vi "MCLScanPSD.vi"(0 "In Image":T1(plugin-control)=refnum, 1 "Trap Detector":dbl[](array[numeric]), 2 "Scan steps (x)":u64, 3 "Scan lines (y)":u64, 4 "Cycles/step (MCL)":u64, 5 "NewScan?":bool) -> (14 "Out Image":T1(plugin-control))   [LabVIEW 2013]
uses:
  <vilib>/Analysis/baseanly.llb/Mean (DBL).vi
  <vilib>/vision/NI_Vision_Development_Module.lvlib
  <vilib>/Analysis/NI_AALBase.lvlib
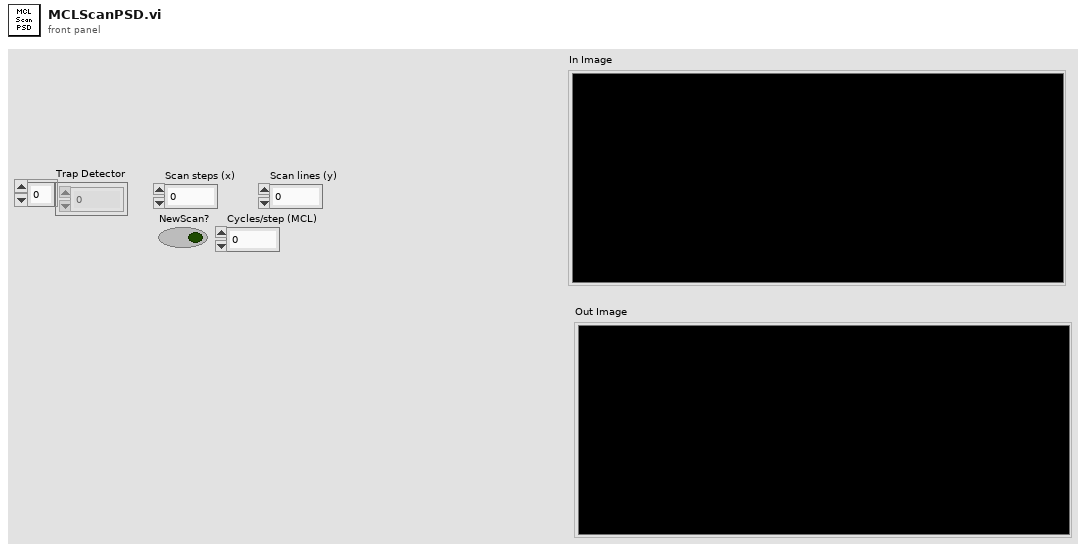
[diagram p1: front panel]
types:
  T1 = typedef "IMAQ Image.ctl" = refnum<image>
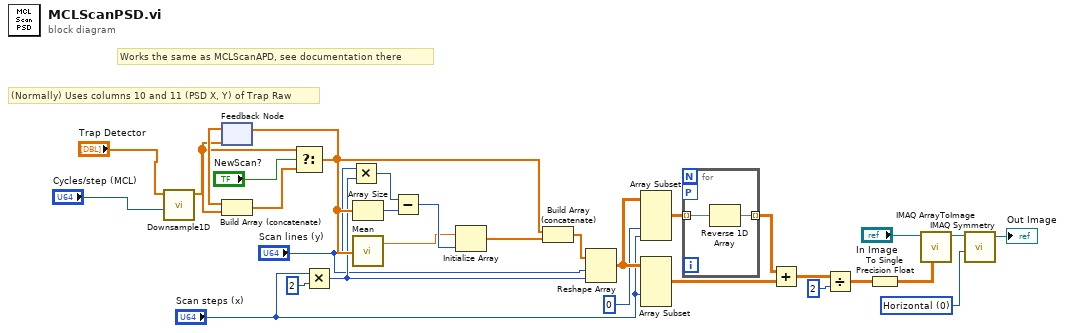
[diagram p0: block diagram]
diagram:
  w27 = u32 0 items=["Horizontal", "Vertical", "Central", "1st Diagonal", "2nd Diagonal"] ("Type of Symmetry")
  # "Works the same as MCLScanAPD, see documentation there"
  # "(Normally) Uses columns 10 and 11 (PSD X, Y) of Trap Raw"
  n1 = call "Downsample1D.vi"("Avg N"="Cycles/step (MCL)", "Array In"="Trap Detector") -> ("Array Out"=w5:dbl[])  [unwired: 9 in]
  n2 = feedback #1(w5) -> (w17:dbl[])
  n3 = Build Array (concatenate)(w17, w5) -> (w18:dbl[])
  n4 = Select(t=w5, s="NewScan?", f=w18) -> (s? t:f=w10:dbl[])
  n5 = feedback-in #1(w10) -> ()
  n6 = Multiply(x="Scan steps (x)", y=2) -> (x*y=w2:u64)
  n7 = Multiply(x="Scan lines (y)", y=w2) -> (x*y=w12:u64)
  n8 = Array Size(array=w10) -> (size(s)=w11:i32)
  n9 = call-poly <vilib>:"Mean.vi"("X"=w10) -> ("mean"=w7:dbl)  [unwired: 1 out]
  n10 = Subtract(x=w12, y=w11) -> (x-y=w9:u64)
  n11 = Initialize Array(w7, w9) -> (w6:dbl[])
  n12 = Build Array (concatenate)(w10, w6) -> (w16:dbl[])
  n13 = Reshape Array(w16, "Scan lines (y)", w2) -> (w25:dbl[][])
  n14 = Array Subset(array=w25, index (col)=0 ("index"), length (col)="Scan steps (x)") -> (w20:dbl[][])  [unwired: 2 in]
  n15 = Array Subset(array=w25, index (col)="Scan steps (x)") -> (w22:dbl[][])  [unwired: 3 in]
  n16 = for {
    tunnel: w20 -> [w32] mode=indexing
    tunnel: [w31] -> w21 mode=indexing
    workers-P: _ -> [_]
    n17 = Reverse 1D Array(array=w32) -> (reversed array=w31:dbl[])
  }
  n18 = Add(x=w21, y=w22) -> (x+y=w23:dbl[][])
  n19 = Divide(x=w23, y=2) -> (x/y=w29:dbl[][])
  n20 = To Single Precision Float(number=w29) -> (single precision float=w28:sgl[][])
  n21 = call "IMAQ ArrayToImage"("Image Pixels (Float)"=w28, "Image"="In Image") -> ("Image Out"=w26:T1)  [unwired: 8 in, 1 out]
  n22 = call "IMAQ Symmetry"("Type of Symmetry"=w27, "Image Src"=w26) -> ("Image Dst Out"=→"Out Image":T1)  [unwired: 3 in, 1 out]
